vi "from string.vi"(8 "error in":errorcluster, 9 "data":string, 10 "version":string, 11 "fixed channel configuration in":refnum<class "ScaleAndLimitModule configuration.lvclass">) -> (0 "error out":errorcluster, 3 "fixed channel configuration out":refnum<class "ScaleAndLimitModule configuration.lvclass">)   [LabVIEW 2017, in "ScaleAndLimitModule configuration.lvclass"]
doc: "Provides an interface for loading a module configuration from a file or other serialized data source. It is recommended that all children of this class store data in two sets--data required for its own initialization, and any data required for parent initialization--and that each implementation uses the <b>Call Parent Method</b> primitive to de-serialize parent information. As a result, it is expected that every module configuration class calls <b>component configuration.lvclass:From String.vi</b>.\nNI Tag Bus Module Framework 1.0.3.43\nNI Systems Engineering"
uses:
  ScaleAndLimitModule configuration.lvclass
  <vilib>/NI/PowerElectronicsControl/ScaleAndLimit/Interface/Configuration.ctl
  ScaleAndLimitModule configuration.lvclass/ScaleAndLimitModule configuration.ctl
  <vilib>/NI/DCAF/Tag Editor Core/control module/configuration/control module configuration.lvclass
  <vilib>/NI/Configuration Framework/serializable configuration/NISE_CEF_serializable configuration.lvclass
  <vilib>/NI/PowerElectronicsControl/ScaleAndLimit/Interface/ScaleAndLimitInterface.lvlib
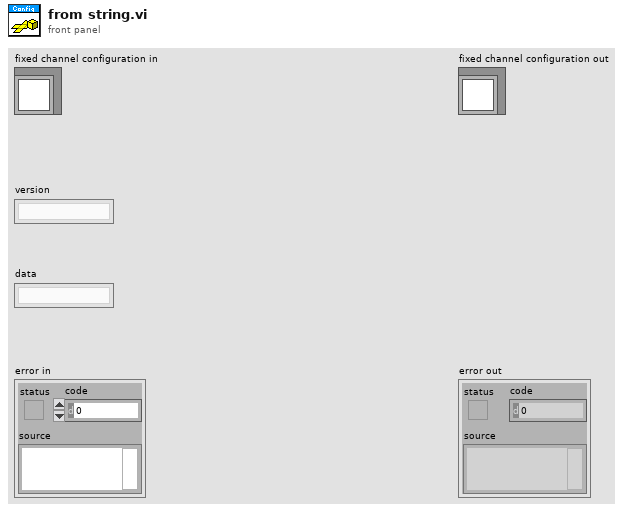
[diagram p1: front panel]
types:
  T1 = typedef "ScaleAndLimitInterface.lvlib/Configuration.ctl" = cluster{"Name":string, "M":dbl, "B":i16, "HighLimit":dbl, "LowLimit":dbl, "LimitsEnabled":bool}
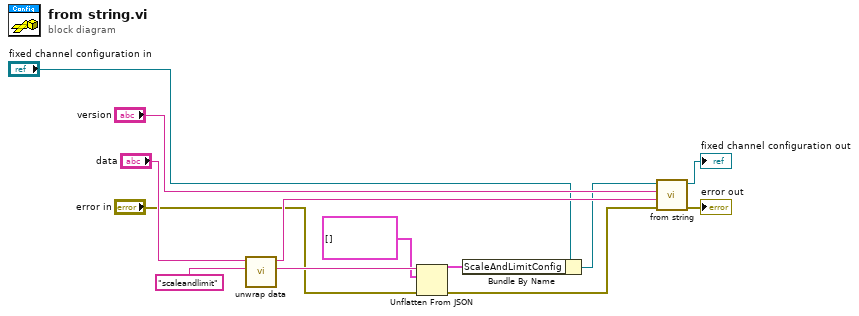
[diagram p0: block diagram]
diagram:
  n1 = call <vilib>:"unwrap data.vi"("identifier"="scaleandlimit", "data to unwrap"="data") -> ("unwrapped data"=w5:string, "remaining string"=w8:string)  [unwired: 8 in]
  n2 = Unflatten From JSON(JSON string=w5, type and defaults=T1[] [] ("ScaleAndLimitConfig"), error in (no error)="error in") -> (value=w2:T1[], error out=w3:errorcluster)  [unwired: 4 in]
  n3 = Bundle By Name(cluster="fixed channel configuration in", "ScaleAndLimitConfig"=w2) -> (w6:refnum<class "ScaleAndLimitModule configuration.lvclass">)
  n4 = call-parent "from string.vi"("error in"=w3, "data"=w8, "version"="version", "fixed channel configuration in"=w6) -> ("error out"=→"error out":errorcluster, "fixed channel configuration out"=→"fixed channel configuration out":refnum<class "ScaleAndLimitModule configuration.lvclass">)  [unwired: 6 in]
